vi "Pendulum Manual.vi"() -> ()   [LabVIEW 2018]
uses:
  Model/Target.ctl
  Model/States.ctl
  <vilib>/Simulation/Scripting/Companion Diagram/SimConfigNode/SimParams.ctl
  <vilib>/Simulation/Scripting/Companion Diagram/SimConfigNode/_simSolvers.ctl
  <vilib>/Simulation/Implementation/Shared/SIMSCR Execution Mode.ctl
  <vilib>/Simulation/Param Hierarchy/Typedefs/SIMPH Param Control Actions.ctl
  <vilib>/Simulation/Implementation/Shared/NILVSim_ParamChanged.vi
  <vilib>/Simulation/Implementation/Shared/NILVSIM_BeginStep.vi
  <vilib>/Simulation/Implementation/Shared/NILVSim_Manager.vi
  <vilib>/Utility/error.llb/Clear Errors.vi
  <vilib>/Simulation/Implementation/Shared/NILVSim_FinalizeModel.vi
  <vilib>/Simulation/Implementation/Shared/SIM Unbundle Sim Info.vi
  <vilib>/Simulation/Implementation/Shared/NILVSim_Initialize.vi
  <vilib>/Simulation/Utility/Implementation/NILVSim Get Time and IsAcceptedStep.vi
  <vilib>/Simulation/Implementation/Shared/SIMSH Read Queue.vi
  <vilib>/Simulation/Implementation/Shared/NILVSim_GetModelError.vi
  <vilib>/Simulation/Implementation/Shared/SIM Bundle Sim Info.vi
  <vilib>/Simulation/Scripting/Companion Diagram/SimConfigNode/SimDog.xnode
  Model/Cart Pendulum Model.vi
  <vilib>/Simulation/Implementation/XNodeFramework/SimXNode/SimX.xnode
  <vilib>/Simulation/Implementation/Shared/NI_SIM_Implementation.lvlib
panel:
  in  "Initial States":T1=[0.0, 0.0, 3.1416, 0.0] format="%.4f"
  out "States":T1 format="%.4f"
  out "Off Track":bool
  out "Done":bool
  out "In Range Seconds":dbl format="%.2f"
  out "In Range?":bool
  in  "Target":T2={"Position"=0.0, "Invert"=TRUE} {"Position" min=-0.5 max=0.5 step=0.1 format="%.2g"}
  out "Seconds":dbl format="%.2f"
  in  "stop":bool
  out "Pendulum":picture
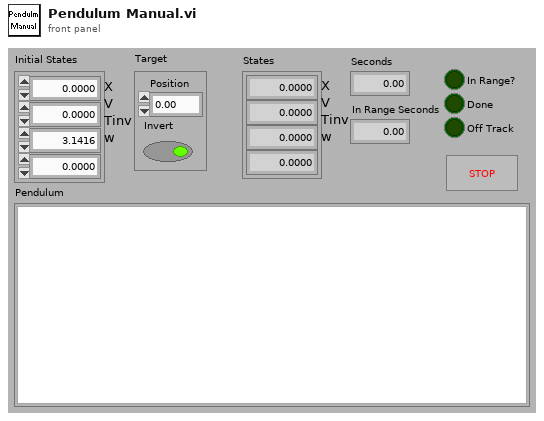
[diagram p1: front panel]
types:
  T1 = typedef "States.ctl" = dbl[]
  T2 = typedef "Target.ctl" = cluster{"Position":dbl, "Invert":bool}
  T3 = typedef "SIMSCR Execution Mode.ctl" = enum16{"Simulate to Completion", "Single Time-Step Simulation (Fixed Step Only)"}
  T4 = typedef "SIMPH Param Control Actions.ctl" = enum16{"get params", "set params"}
  T5 = cluster{"SIMSH Sim Time":dbl, "Integrator 3":cluster{"output":dbl[]}, "Build Array":cluster{"appended array":dbl[]}, "Index Array":cluster{"element":dbl}, "Negate 2":cluster{"-x":dbl}, "Negate":cluster{"-x":dbl}, "Sine & Cosine":cluster{"sin(x)":dbl, "cos(x)":dbl}, "Formula Node":cluster{"dx":dbl, "ddx":dbl, "dT":dbl, "ddT":dbl}}
  T6 = typedef "SimParams.ctl" = cluster{"Initial Time (s)":dbl, "Final Time (s)":dbl, "Step Size (s)":dbl, "ODE Solver":T7, "Minimum Step Size (s)":dbl, "Maximum Step Size (s)":dbl, "Relative Tolerance":dbl, "Absolute Tolerance":dbl, "Software Timing":bool, "Initial Step Size (s)":dbl, "Automatic Fixed Step Size?":bool, "Automatic Discrete Step Size?":bool, "Discrete Step Size (s)":dbl, "Calculate using Time Step":bool, "Solver Wired?":bool, "Prev.Frm.Expected End":u64, "Prev.Frm.Actual End":u64, "Prev.Frm.Finished Late?":bool, "Prev.Iter.Expected End":u64, "Prev.Iter.Actual End":u64, "Prev.Iter.Finished Late?":bool, "Expected Iteration Start":u64, "Actual Iteration Start":u64, "Expected Frame Start":u64, "Actual Frame Start":u64, "Source Name":string, "Name":string, "Period":i64, "Deadline":i64, "Offset":i64, "Start":i64, "Priority":i32, "Timeout":i32, "Processor":i32, "Mode":enum32{"No Change", "Process missed periods, maintain original phase", "Discard missed periods, maintain original phase", "Process missed periods, ignore original phase", "Discard missed periods, ignore original phase"}, "Wakeup reason":enum32{"Normal", "Aborted", "Asynchronous wakeup", "Timing source error", "Timed loop error", "Timeout"}, "Error":errorcluster, "Source Type":string, "Secondary Source Type":string, "Global End Time":u64, "Global Start Time":u64, "Full Solver Reset":bool, "Execution Mode":T3, "Nan/Inf Check":bool, "Custom Solver Library":string, "Solver Is Variable":bool, "custom solver name":string, "Signal Collection Decimation":u32}
  T7 = typedef "_simSolvers.ctl" = enum16{"Runge-Kutta 1 (Euler)", "Runge-Kutta 2", "Runge-Kutta 3", "Runge-Kutta 4", "Runge-Kutta 23 (variable)", "Runge-Kutta 45 (variable)", "BDF (variable)", "Adams-Moulton (variable)", "Rosenbrock (variable)", "Discrete States Only", "SDIRK 4 (variable)", "Radau 5 (variable)", "Radau 9 (variable)", "Radau 13 (variable)", "Radau [Variable Order] (variable)", "Gear's Method (variable)", "Linearizer", "State Query", "Trim Eval", "Custom Solver"}
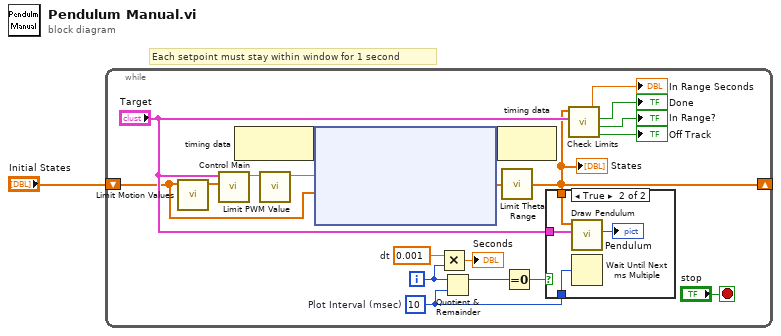
[diagram p0: block diagram]
diagram:
  # "Each setpoint must stay within window for 1 second"
  n1 = while {
    shift-right: [w3] -> _
    shift-left: "Initial States" -> [w6]
    i -> [w18]
    stop <- "stop" stop-if-true
    w10 = 0.001  # dt
    w11 = u32 10  # Plot Interval (msec)
    n2 = call "Limit Motion Values.vi"("States In"=w6) -> ("States Out"=w9:T1)  [unwired: 10 in]
    n3 = call "Control Main.vi"("States"=w9, "Target"="Target") -> ("PWM"=w5:dbl)  [unwired: 9 in]
    n4 = node-c288() -> (w8:variant)  [unwired: 1 in]
    n5 = call "Limit PWM Value.vi"("PWM In"=w5) -> ("PWM Out"=w4:dbl)  [unwired: 10 in]
    n6 = node-c254 ("Control & Simulation Loop 2")(w8, w4, w6) -> (w7:variant, w2:dbl[])
    n7 = Multiply(x=w10, y=w18) -> (x*y=→"Seconds":dbl)
    n8 = Quotient & Remainder(x=w18, y=w11) -> (x-y*floor(x/y)=w21:u32)  [unwired: 1 out]
    n9 = node-c288(w7) -> ()  [unwired: 1 out]
    n10 = call "Limit Theta Range.vi"("States In"=w2) -> ("States Out"=w3:T1)
    "States" <- w3
    n11 = Equal To 0?(x=w21) -> (x = 0?=w20:bool)
    n12 = case shown="True" w20 {
      tunnel: w3 -> [_ w257]
      tunnel: "Target" -> [_ w256]
      tunnel: w11 -> [_ w255]
      frame False {
      }
      frame True {
        n13 = call "Draw Pendulum.vi"("Target"=w256, "States In"=w257) -> ("Picture"=→"Pendulum":picture)  [unwired: 1 in, 8 out]
        n14 = Wait Until Next ms Multiple(millisecond multiple=w255) -> ()  [unwired: 1 out]
      }
    }
    n15 = call "Check Limits.vi"("Target"="Target", "States"=w3) -> ("Off Track"=→"Off Track":bool, "In Range"=→"In Range?":bool, "Done"=→"Done":bool, "In Range Seconds"=→"In Range Seconds":dbl)  [unwired: 3 in]
  }
